vi "Elliptec.vi"() -> ()   [LabVIEW 2015]
doc: "串口助手V1.0\n作者：资道周\nzidaozhou@163.com"
uses:
  <vilib>/Instr/_visa.llb/VISA Configure Serial Port (Instr).vi
panel:
  out "ERROR":bool
  out "x/y":dbl
  in  "Point":bool
  out "VISA resource name out":refnum<visa-resource-name>
  out "error out":errorcluster
  out "布尔":bool
  in  "发送数据":bool
  in  "open":bool
  in  "?":dbl
  in  "串   口":T1(ring)
  # "Absolute"
  # "mm"
  # "25mm"
  # "0mm"
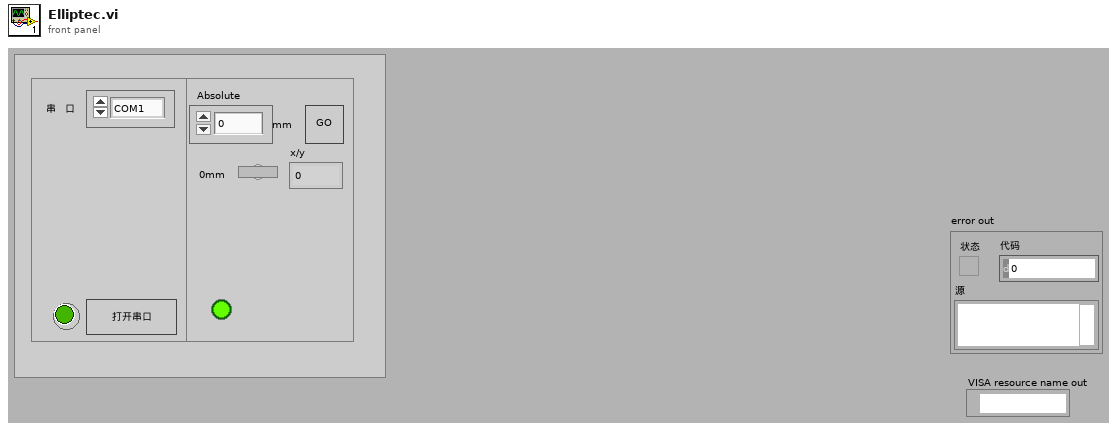
[diagram p1: front panel]
types:
  T1 = enum16{"COM1", "COM2", "COM3", "COM4", "COM5", "COM6"}
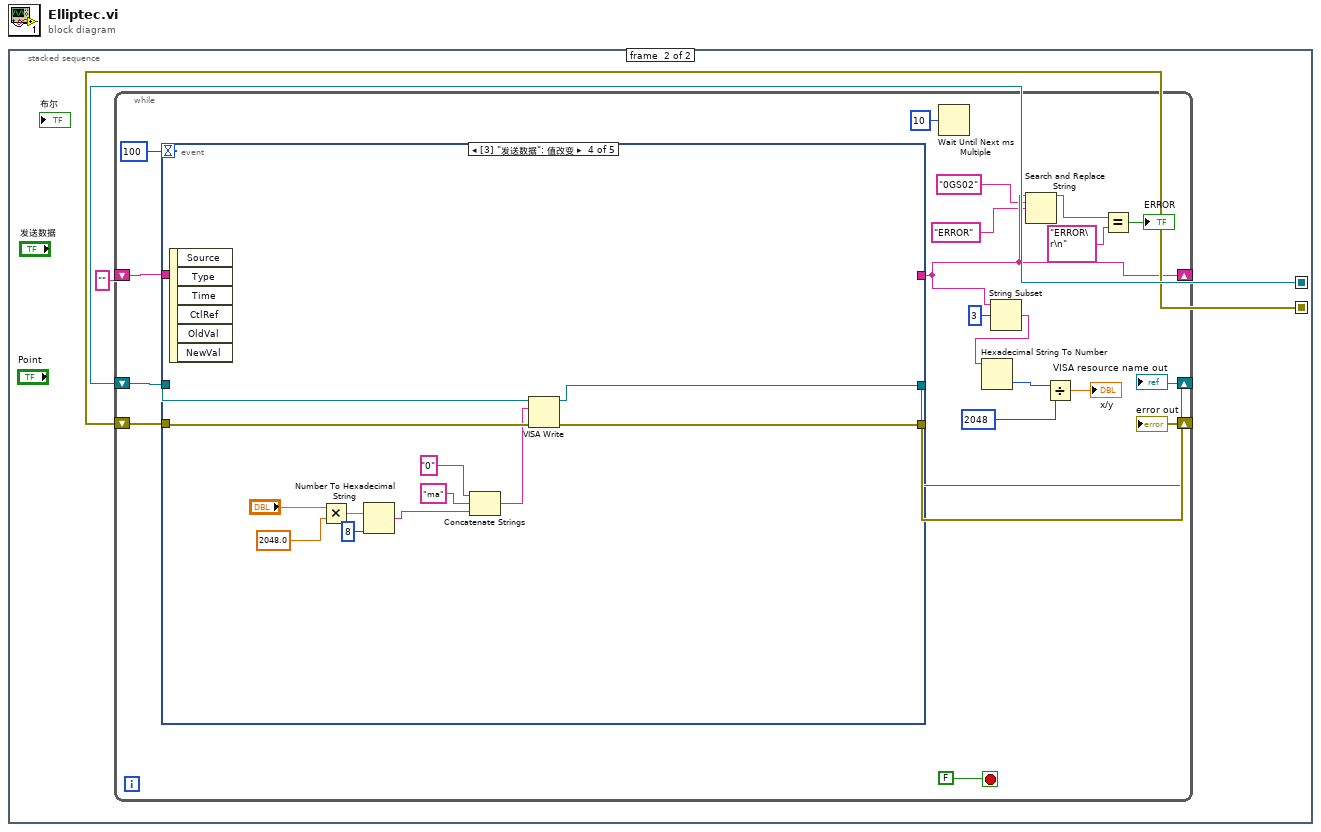
[diagram p0: block diagram]
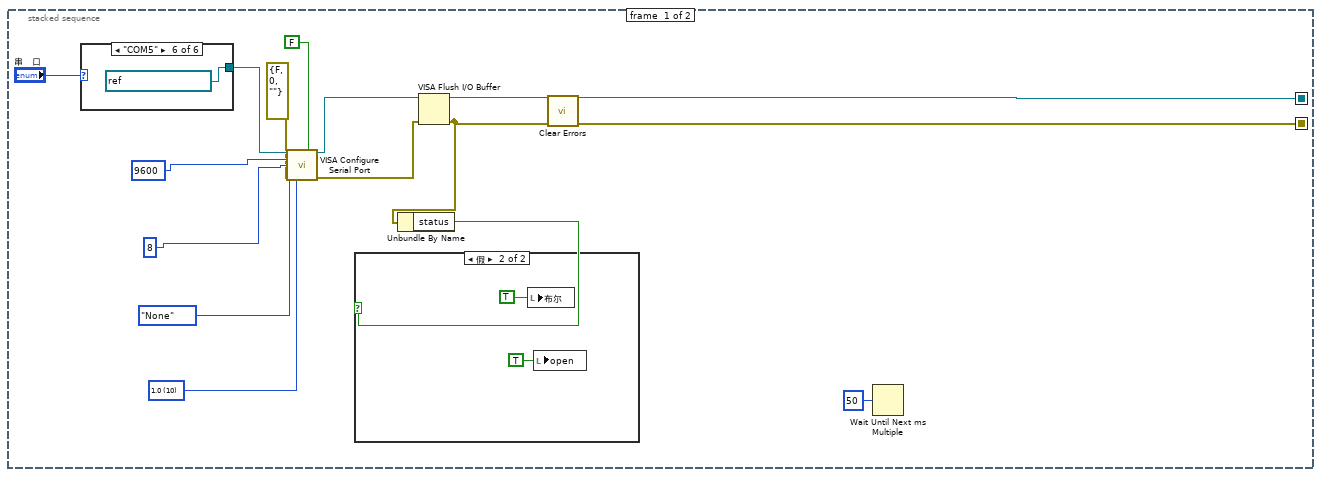
[diagram p2: hidden frame]
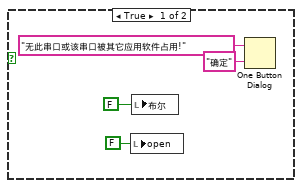
[diagram p3: hidden frame]
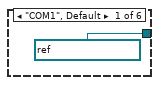
[diagram p4: hidden frame]
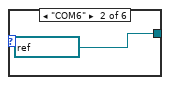
[diagram p5: hidden frame]
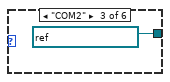
[diagram p6: hidden frame]
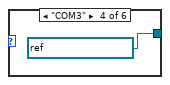
[diagram p7: hidden frame]
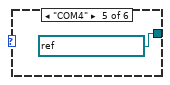
[diagram p8: hidden frame]
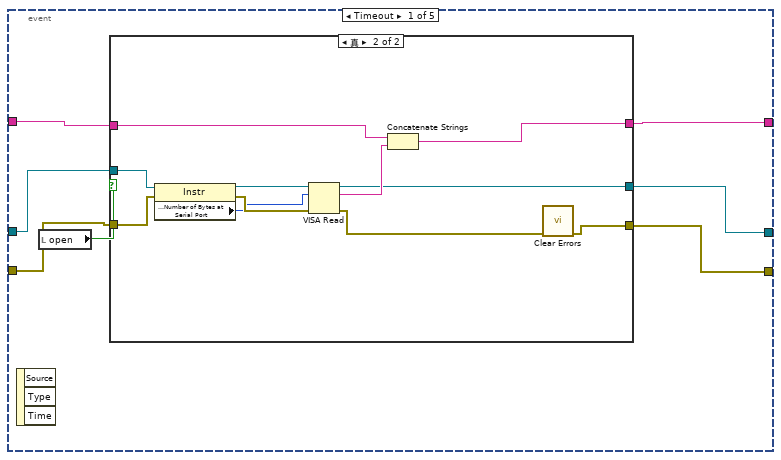
[diagram p9: hidden frame]
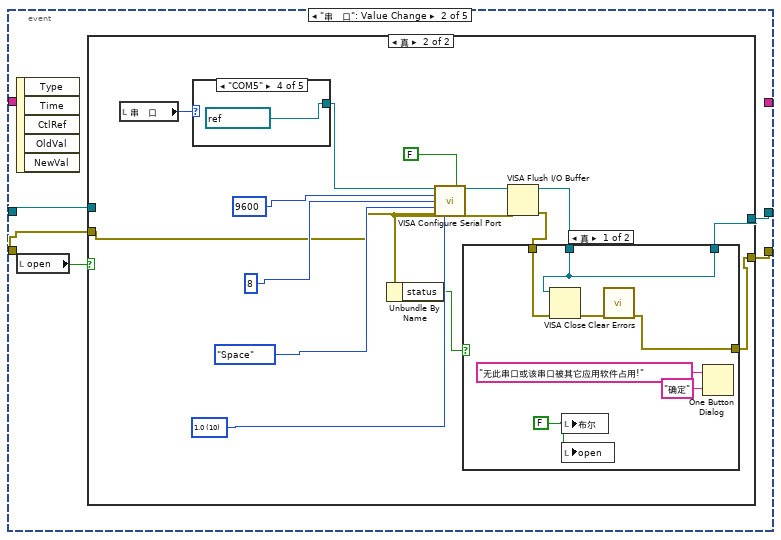
[diagram p11: hidden frame]
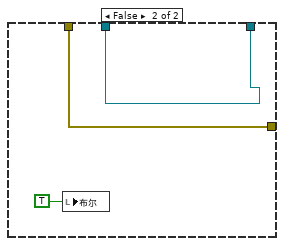
[diagram p13: hidden frame]
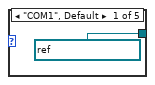
[diagram p14: hidden frame]
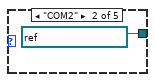
[diagram p15: hidden frame]
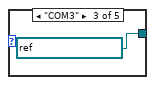
[diagram p16: hidden frame]
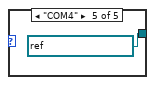
[diagram p17: hidden frame]
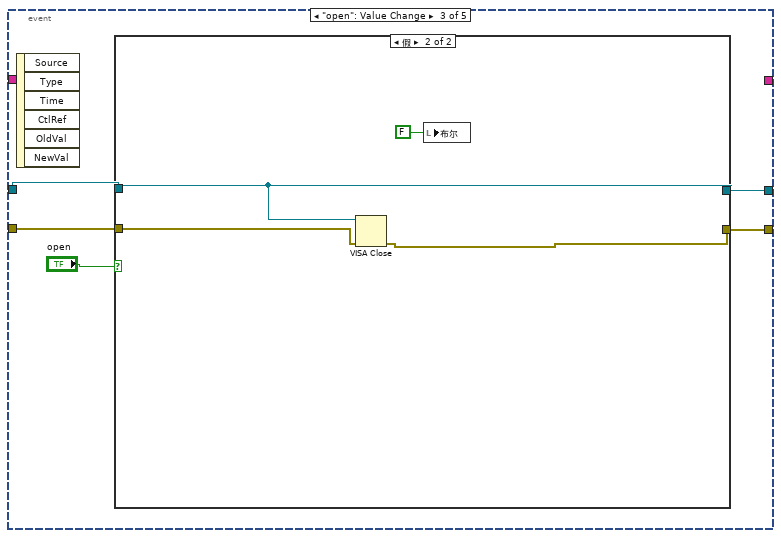
[diagram p18: hidden frame]
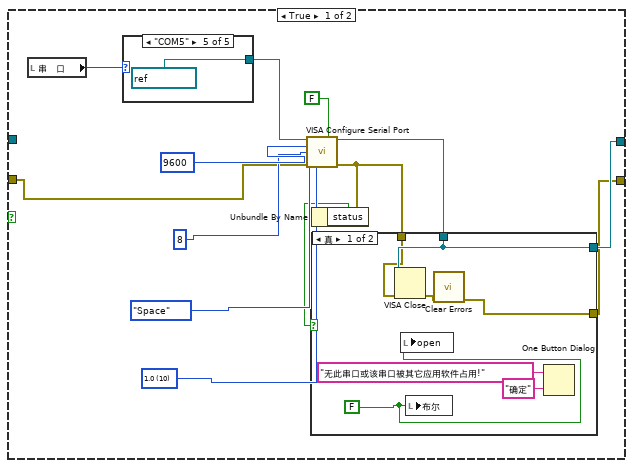
[diagram p19: hidden frame]
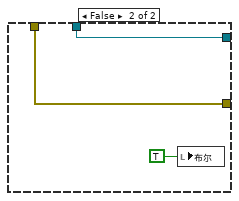
[diagram p20: hidden frame]
diagram:
  n1 = stacked-sequence {
    seq-local: [w4 _] -> [_ w31]
    seq-local: [w3 _] -> [_ w30]
    frame #0 {
      w9 = u16 10 items=["1.0"=10, "1.5"=15, "2.0"=20] ("stop bits (10: 1 bit)")
      n2 = case shown="\"COM5\"" "串   口" {
        tunnel: [refnum<visa-resource-name> "ASRL1::INSTR" ("串口：") refnum<visa-resource-name> "COM5" ("串口：") refnum<visa-resource-name> "ASRL2::INSTR" ("串口：") refnum<visa-resource-name> "ASRL3::INSTR" ("串口：") refnum<visa-resource-name> "ASRL4::INSTR" ("串口：") refnum<visa-resource-name> "ASRL5::INSTR" ("串口：")] -> w15
        frame "COM1", Default {
        }
        frame "COM6" {
        }
        frame "COM2" {
        }
        frame "COM3" {
        }
        frame "COM4" {
        }
        frame "COM5" {
        }
      }
      n3 = call-poly "VISA Configure Serial Port"("VISA resource name"=w15, "Enable Termination\nChar (T)"=FALSE ("Enable Termination\nChar (T)"), "baud rate (9600)"=u32 9600, "data bits (8)"=u16 8, "parity (0:none)"=enum16{"None", "Odd", "Even", "Mark", "Space"}."None", "error in (no error)"=errorcluster {"status"=FALSE, "code"=0, "source"=""}, "stop bits (10: 1 bit)"=w9) -> ("VISA resource name out"=w6:refnum<visa-resource-name>, "error out"=w5:errorcluster)  [unwired: 1 in, 6 out]
      n4 = VISA Flush I/O Buffer(VISA resource name=w6, error in (no error)=w5) -> (VISA resource name out=w4:refnum<visa-resource-name>, error out=w2:errorcluster)  [unwired: 1 out]
      n5 = Unbundle By Name(w2) -> ("status"=w7:bool)
      n6 = case shown="假" w7 {
        frame True {
          n7 = local write "open"(FALSE ("open")) -> ()
          n8 = local write "布尔"(FALSE ("布尔")) -> ()
          n9 = One Button Dialog(message="无此串口或该串口被其它应用软件占用!" ("消息"), button name ("OK")="确定" ("按钮名称（“确定”）")) -> ()  [unwired: 1 out]
        }
        frame False {
          n10 = local write "布尔"(TRUE ("布尔")) -> ()
          n11 = local write "open"(TRUE ("open")) -> ()
        }
      }
      n12 = call <vilib>:"Clear Errors.vi"("error in (no error)"=w2) -> ("error out"=w3:errorcluster)  [unwired: 1 in, 5 out]
      n13 = Wait Until Next ms Multiple(millisecond multiple=u32 50 ("毫秒倍数")) -> ()  [unwired: 1 out]
    }
    frame #1 {
      n14 = while {
        shift-right: [w47] -> w32
        shift-left: w30 -> [w48]
        shift-right: [w46] -> w29
        shift-left: w31 -> [w45]
        shift-right: [w38] -> _
        shift-left: "" -> [w44]
        stop <- FALSE stop-if-true
        n15 = event shown="[3] \"发送数据\": 值改变" {
          selector: _ -> [_ _ _ _ _]
          dyn-events: _ -> [_ _ _ _ _]
          timeout: 100 -> [_ _ _ _ _]
          tunnel: [w57 w77 w113 w155 w160] -> w47
          tunnel: w48 -> [w58 w74 w112 w157 w162]
          tunnel: [w56 w76 w111 w156 w161] -> w46
          tunnel: w45 -> [w55 w75 w110 w158 w163]
          tunnel: w44 -> [w53 _ _ _ _]
          tunnel: [w52 _ _ _ _] -> w38
          event Timeout {
            n16 = event-data() -> ()  [unwired: 4 out]
            n17 = local read "open"() -> (w54:bool)
            n18 = case shown="真" w54 {
              tunnel: w58 -> [w60 w69]
              tunnel: [w60 w64] -> w57
              tunnel: [w61 w68] -> w56
              tunnel: w55 -> [w61 w67]
              tunnel: w53 -> [w59 w63]
              tunnel: [w59 w62] -> w52
              frame False {
              }
              frame True {
                n19 = property class="Instr"(reference=w67, error in=w69) -> (reference out=w72:refnum<visa-resource-name>, error out=w71:errorcluster, "Serial Settings:Number of Bytes at Serial Port"=w66:u32)
                n20 = VISA Read(VISA resource name=w72, byte count=w66, error in (no error)=w71) -> (VISA resource name out=w68:refnum<visa-resource-name>, read buffer=w70:string, error out=w65:errorcluster)  [unwired: 1 out]
                n21 = Concatenate Strings(w63, w70) -> (w62:string)
                n22 = call <vilib>:"Clear Errors.vi"("error in (no error)"=w65) -> ("error out"=w64:errorcluster)  [unwired: 1 in, 5 out]
              }
            }
          }
          event "串   口": Value Change {
            n23 = event-data() -> ()  [unwired: 6 out]
            n24 = local read "open"() -> (w73:bool)
            n25 = case shown="真" w73 {
              tunnel: [w78 w80] -> w77
              tunnel: [w79 w81] -> w76
              tunnel: w75 -> [w79 _]
              tunnel: w74 -> [w78 w84]
              frame False {
              }
              frame True {
                w90 = u16 10 items=["1.0"=10, "1.5"=15, "2.0"=20] ("stop bits (10: 1 bit)")
                n26 = local read "串   口"() -> (w94:T1)
                n27 = case shown="\"COM5\"" w94 {
                  tunnel: [refnum<visa-resource-name> "ASRL1::INSTR" ("串口：") refnum<visa-resource-name> "ASRL2::INSTR" ("串口：") refnum<visa-resource-name> "ASRL3::INSTR" ("串口：") refnum<visa-resource-name> "COM5" ("串口：") refnum<visa-resource-name> "ASRL4::INSTR" ("串口：")] -> w89
                  frame "COM1", Default {
                  }
                  frame "COM2" {
                  }
                  frame "COM3" {
                  }
                  frame "COM5" {
                  }
                  frame "COM4" {
                  }
                }
                n28 = call-poly "VISA Configure Serial Port"("VISA resource name"=w89, "Enable Termination\nChar (T)"=FALSE ("Enable Termination\nChar (T)"), "baud rate (9600)"=u32 9600, "data bits (8)"=u16 8, "parity (0:none)"=enum16{"None", "Odd", "Even", "Mark", "Space"}."Space", "error in (no error)"=w84, "stop bits (10: 1 bit)"=w90) -> ("VISA resource name out"=w86:refnum<visa-resource-name>, "error out"=w85:errorcluster)  [unwired: 1 in, 6 out]
                n29 = Unbundle By Name(w85) -> ("status"=w87:bool)
                n30 = VISA Flush I/O Buffer(VISA resource name=w86, error in (no error)=w85) -> (VISA resource name out=w82:refnum<visa-resource-name>, error out=w83:errorcluster)  [unwired: 1 out]
                n31 = case shown="真" w87 {
                  tunnel: w83 -> [w98 w102]
                  tunnel: w82 -> [w99 w103]
                  tunnel: [w99 w103] -> w81
                  tunnel: [w95 w102] -> w80
                  frame True {
                    w97 = FALSE ("布尔")
                    n32 = VISA Close(VISA resource name=w99, error in (no error)=w98) -> (error out=w96:errorcluster)
                    n33 = local write "布尔"(w97) -> ()
                    n34 = local write "open"(w97) -> ()
                    n35 = call <vilib>:"Clear Errors.vi"("error in (no error)"=w96) -> ("error out"=w95:errorcluster)  [unwired: 1 in, 5 out]
                    n36 = One Button Dialog(message="无此串口或该串口被其它应用软件占用!" ("消息"), button name ("OK")="确定" ("按钮名称（“确定”）")) -> ()  [unwired: 1 out]
                  }
                  frame False {
                    n37 = local write "布尔"(TRUE ("布尔")) -> ()
                  }
                }
              }
            }
          }
          event "open": Value Change {
            n38 = event-data() -> ()  [unwired: 7 out]
            n39 = case shown="假" "open" {
              tunnel: [w117 w144] -> w113
              tunnel: w112 -> [w119 w145]
              tunnel: [w118 w143] -> w111
              tunnel: w110 -> [_ w143]
              frame True {
                w121 = u16 10 items=["1.0"=10, "1.5"=15, "2.0"=20] ("stop bits (10: 1 bit)")
                n40 = local read "串   口"() -> (w127:T1)
                n41 = case shown="\"COM5\"" w127 {
                  tunnel: [refnum<visa-resource-name> "ASRL1::INSTR" ("串口：") refnum<visa-resource-name> "ASRL2::INSTR" ("串口：") refnum<visa-resource-name> "ASRL3::INSTR" ("串口：") refnum<visa-resource-name> "ASRL4::INSTR" ("串口：") refnum<visa-resource-name> "COM5" ("串口：")] -> w126
                  frame "COM1", Default {
                  }
                  frame "COM2" {
                  }
                  frame "COM3" {
                  }
                  frame "COM4" {
                  }
                  frame "COM5" {
                  }
                }
                n42 = call-poly "VISA Configure Serial Port"("VISA resource name"=w126, "Enable Termination\nChar (T)"=FALSE ("Enable Termination\nChar (T)"), "baud rate (9600)"=u32 9600, "data bits (8)"=u16 8, "parity (0:none)"=enum16{"None", "Odd", "Even", "Mark", "Space"}."Space", "error in (no error)"=w119, "stop bits (10: 1 bit)"=w121) -> ("VISA resource name out"=w116:refnum<visa-resource-name>, "error out"=w115:errorcluster)  [unwired: 1 in, 6 out]
                n43 = Unbundle By Name(w115) -> ("status"=w120:bool)
                n44 = case shown="真" w120 {
                  tunnel: w115 -> [w130 w135]
                  tunnel: w116 -> [w131 w136]
                  tunnel: [w131 w136] -> w118
                  tunnel: [w128 w135] -> w117
                  frame True {
                    w132 = FALSE ("布尔")
                    n45 = VISA Close(VISA resource name=w131, error in (no error)=w130) -> (error out=w129:errorcluster)
                    n46 = local write "open"(w132) -> ()
                    n47 = local write "布尔"(w132) -> ()
                    n48 = call <vilib>:"Clear Errors.vi"("error in (no error)"=w129) -> ("error out"=w128:errorcluster)  [unwired: 1 in, 5 out]
                    n49 = One Button Dialog(message="无此串口或该串口被其它应用软件占用!" ("消息"), button name ("OK")="确定" ("按钮名称（“确定”）")) -> ()  [unwired: 1 out]
                  }
                  frame False {
                    n50 = local write "布尔"(TRUE ("布尔")) -> ()
                  }
                }
              }
              frame False {
                n51 = VISA Close(VISA resource name=w143, error in (no error)=w145) -> (error out=w144:errorcluster)
                n52 = local write "布尔"(FALSE ("布尔")) -> ()
              }
            }
          }
          event "发送数据": Value Change {
            n53 = event-data() -> ()  [unwired: 7 out]
            n54 = Multiply(x="?", y=2048.0) -> (x*y=w153:dbl)
            n55 = Number To Hexadecimal String(1:i16 8 ("宽度(-)"), 2:w153) -> (0:w149:string)
            n56 = Concatenate Strings("0" ("写入缓冲区"), "ma" ("字符串"), w149) -> (w148:string)
            n57 = VISA Write(VISA resource name=w158, write buffer=w148, error in (no error)=w157) -> (VISA resource name out=w156:refnum<visa-resource-name>, error out=w155:errorcluster)  [unwired: 1 out]
          }
          event "Point": Value Change {
            n58 = event-data() -> ()  [unwired: 7 out]
            n59 = local read "Point"() -> (w159:bool)
            n60 = case shown="真" w159 {
              tunnel: w163 -> [w168 w181]
              tunnel: w162 -> [w167 w180]
              tunnel: [w165 w179] -> w160
              tunnel: [w166 w178] -> w161
              frame False {
                n61 = Multiply(x=0.0, y=2048.0) -> (x*y=w171:dbl)
                n62 = Number To Hexadecimal String(1:i16 8 ("宽度(-)"), 2:w171) -> (0:w170:string)
                n63 = Concatenate Strings("0" ("写入缓冲区"), "ma" ("字符串"), w170) -> (w175:string)
                n64 = VISA Write(VISA resource name=w168, write buffer=w175, error in (no error)=w167) -> (VISA resource name out=w166:refnum<visa-resource-name>, error out=w165:errorcluster)  [unwired: 1 out]
              }
              frame True {
                n65 = Multiply(x=25.0, y=2048.0) -> (x*y=w183:dbl)
                n66 = Number To Hexadecimal String(1:i16 8 ("宽度(-)"), 2:w183) -> (0:w182:string)
                n67 = Concatenate Strings("0" ("写入缓冲区"), "ma" ("字符串"), w182) -> (w187:string)
                n68 = VISA Write(VISA resource name=w181, write buffer=w187, error in (no error)=w180) -> (VISA resource name out=w178:refnum<visa-resource-name>, error out=w179:errorcluster)  [unwired: 1 out]
              }
            }
          }
        }
        n69 = Wait Until Next ms Multiple(millisecond multiple=u32 10 ("毫秒倍数")) -> ()  [unwired: 1 out]
        n70 = String Subset(string=w38, offset (0)=3 ("偏移量(0)")) -> (substring=w39:string)  [unwired: 1 in]
        n71 = Hexadecimal String To Number(string=w39) -> (number=w43:u32)  [unwired: 2 in, 1 out]
        n72 = Search and Replace String(input string=w38, search string="0GS02" ("搜索字符串"), replace string="ERROR" ("替换字符串(\"\")")) -> (result string=w34:string)  [unwired: 5 in, 3 out]
        n73 = Divide(x=w43, y=u32 2048) -> (x/y=→"x/y":dbl)
        n74 = Equal?(x=w34, y="ERROR\r\n") -> (x = y?=→"ERROR":bool)
      }
      "error out" <- w32
      "VISA resource name out" <- w29
    }
  }
